vi "OAT Polar PG scale.vi"(0 "picture":picture, 1 "desired font(Application)":T2(ring)=enum."Application Font", 2 "decade specs":cluster{"radius":i16, "label":string}[](array[cluster]), 3 "grid measurements":T1 {"end angle" format="%.2f"; "start angle" format="%.2f"; "scale factors"."b" format="%.2f"; "scale factors"."a" format="%.2f"}, 5 "[user-specified font]":T3) -> (6 "new picture":picture)   [LabVIEW 2017]
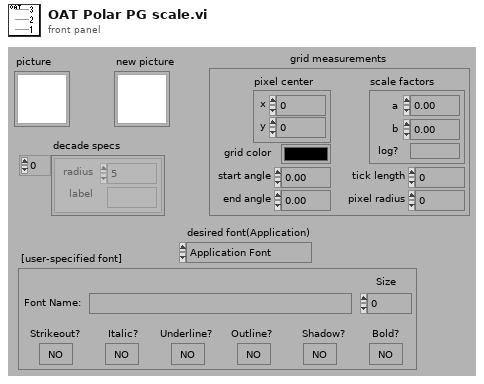
[diagram p1: front panel]
types:
  T1 = cluster{"pixel center":cluster{"x":i16, "y":i16}, "scale factors":cluster{"a":dbl, "b":dbl, "log?":bool}, "grid color":u32, "start angle":dbl, "end angle":dbl, "tick length":i16, "pixel radius":i32}
  T2 = enum16{"User-specified Font", "Application Font", "System Font", "Dialog Font"}
  T3 = cluster{"Font Name:":string, "Size":i16, "Strikeout?":bool, "Italic?":bool, "Underline?":bool, "Outline?":bool, "Shadow?":bool, "Bold?":bool}
  T4 = cluster{bool, bool, bool, "Shadow":u32, "grid color":u32}
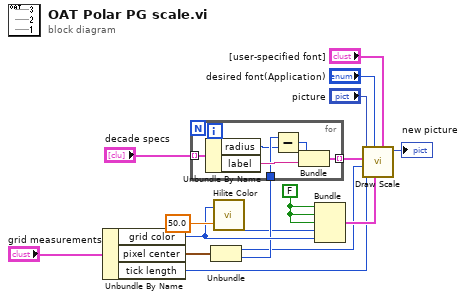
[diagram p0: block diagram]
diagram:
  w6 = FALSE
  n1 = Unbundle By Name("grid measurements") -> ("grid color"=w7:u32, "pixel center"=w5:cluster{"x":i16, "y":i16}, "tick length"=w1:i16)
  n2 = Unbundle(w5) -> ("x"=w3:i16, "y"=w4:i16)
  n3 = for {
    tunnel: "decade specs" -> [w22] mode=indexing
    tunnel: w4 -> [w20]
    tunnel: [w17] -> w11 mode=indexing
    n4 = Unbundle By Name(w22) -> ("radius"=w19:i16, "label"=w21:string)
    n5 = Subtract(x=w20, y=w19) -> (x-y=w18:i16)
    n6 = Bundle(w18, "label"=w21) -> (w17:cluster{i16, "label":string})  [unwired: 1 in]
  }
  n7 = call <vilib>:"Hilite Color.vi"("Percentage(30)"=50.0, "Color In"=w7) -> ("Shadow"=w2:u32)  [unwired: 1 out]
  n8 = Bundle(w6, w6, w6, "Shadow"=w2, "grid color"=w7) -> (w13:T4)  [unwired: 1 in]
  n9 = call <vilib>:"Draw Scale.vi"("[user-specified font]"="[user-specified font]", "scale attributes"=w13, "desired font(Application)"="desired font(Application)", "tick length(3)"=w1, "constant coordinate"=w3, "scale specs"=w11, "picture"="picture") -> ("new picture"=→"new picture":picture)  [unwired: 4 in]
